vi "GOMDBTS2048 integral Set Az Specific.vi"(8 "error in (no error)":errorcluster, 10 "az":dbl, 11 "handle":i32) -> (0 "error out":errorcluster, 3 "function return":i32)   [LabVIEW 2015, in "GOMDBTS2048.lvlib"]
doc: "GOBTS2048DLL int __stdcall GOMDBTS2048_integralSetAzSpecific(int handle, double az);"
uses:
  GOMDBTS2048.lvlib
  runtime/GOMDBTS2048.dll
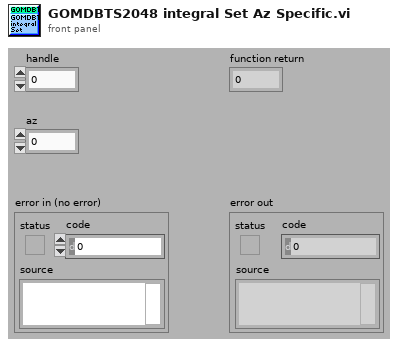
[diagram p1: front panel]
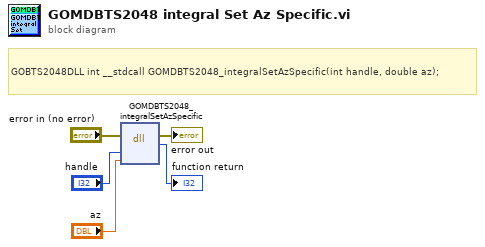
[diagram p0: block diagram]
diagram:
  # "GOBTS2048DLL int __stdcall GOMDBTS2048_integralSetAzSpecific(int handle, double az);"
  n1 = dll-call lib="C:/Users/rkoch/Documents/GO_Library/runtime/GOMDBTS2048.*" fn="GOMDBTS2048_integralSetAzSpecific"(error in="error in (no error)", "handle"="handle", "az"="az") -> (error out=→"error out":errorcluster, →"function return":i32)  [unwired: 4 in, 1 out]
